vi "4bmilo2.vi"() -> ()   [LabVIEW 2010]
uses:
  <vilib>/express/express arith-compare/Formula/XNode/ExpressFormulaBlockNode.xnode
  <vilib>/express/express shared/transition.llb/Dynamic To Waveform Array.vi
  <vilib>/express/express shared/transition.llb/Waveform Array To Dynamic.vi
  <vilib>/express/express arith-compare/Formula/Block/exnFormulaBlock how many pts in the wave.vi
  <vilib>/express/express shared/ex_Modify Signal Name.vi
panel:
  out "au = f(f)":cluster{"Y":dbl[], "Y":dbl[]}[](graph)
  out "Uin, Uout =f(T)":dynamicdata(graph) caption="Uin, Uout = f(t)"
  in  "stop":bool
  out "au(dB)":dbl
  out "Au":dbl
  out "Frekvence":dbl
  out "Uin":dbl
  out "Uout":dbl
  # "Snímaè frekvenèních charakteristik"
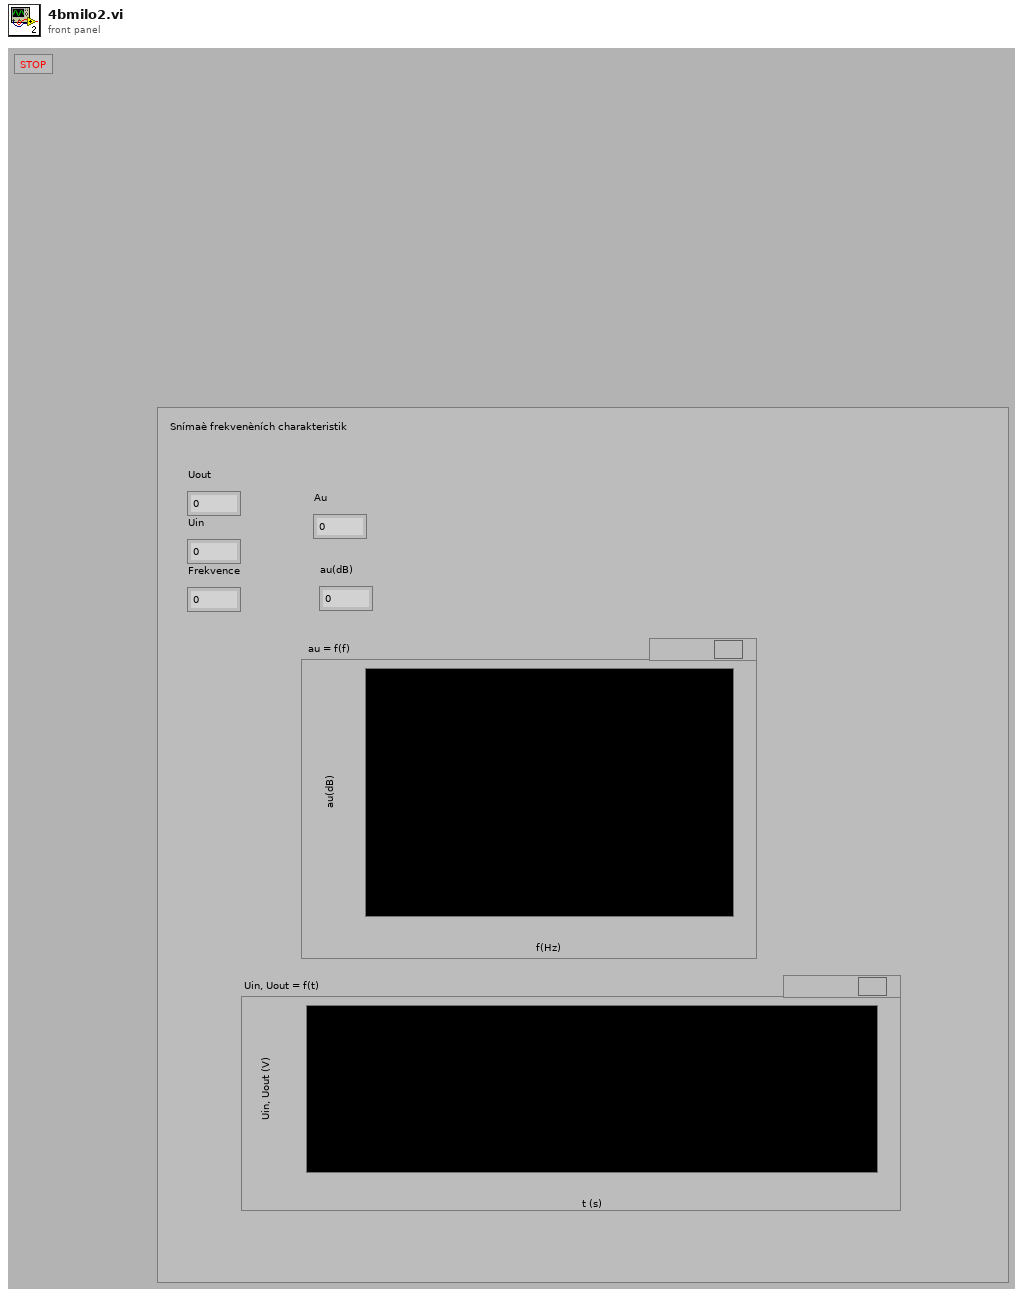
[diagram p1: front panel]
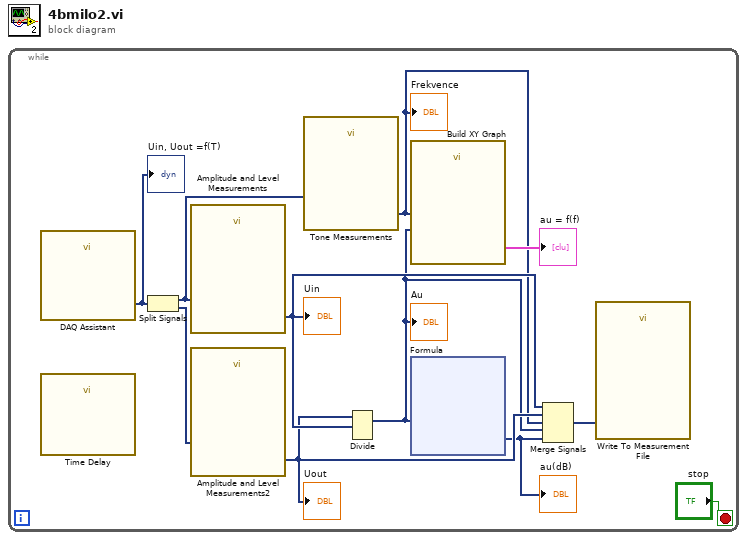
[diagram p0: block diagram]
diagram:
  n1 = while {
    stop <- "stop" stop-if-true
    n2 = call "DAQ Assistant"() -> ("data"=w11:dynamicdata)  [unwired: 17 in, 2 out]
    "Uin, Uout =f(T)" <- w11
    n3 = call "Time Delay"() -> ()  [unwired: 11 in, 1 out]
    n4 = Split Signals(w11) -> (w9:dynamicdata, w10:dynamicdata)  [unwired: 2 in]
    n5 = call "Amplitude and Level Measurements"("Signals"=w9) -> ("RMS"=w5:dynamicdata)  [unwired: 13 in, 1 out]
    "Uin" <- w5
    n6 = call "Amplitude and Level Measurements2"("Signals"=w10) -> ("RMS"=w4:dynamicdata)  [unwired: 13 in, 1 out]
    "Uout" <- w4
    n7 = call "Tone Measurements"("Signals"=w9) -> ("Frequency"=w3:dynamicdata)  [unwired: 9 in, 1 out]
    "Frekvence" <- w3
    n8 = Divide(1:w5, 2:w4) -> (0:w2:dynamicdata)  [unwired: 1 in, 1 out]
    "Au" <- w2
    n9 = call "Build XY Graph"("Y Input"=w2, "X Input"=w3) -> ("XY Graph"=→"au = f(f)":cluster{"Y":dbl[], "Y":dbl[]}[])  [unwired: 3 in, 6 out]
    n10 = xnode "Formula"("Au"=w2) -> ("Result"=w1:dynamicdata)  [unwired: 1 in, 1 out]
    "au(dB)" <- w1
    n11 = Merge Signals(w5, w4, w3, w2, w1) -> (w6:dynamicdata)
    n12 = call "Write To Measurement File"("Signals"=w6) -> ()  [unwired: 16 in, 3 out]
  }
